vi "Get Parameter.vi"(8 "error in (no error)":errorcluster, 11 "SolarSystems M266 in":refnum<class "SolarSystems M266.lvclass">) -> (0 "error out":errorcluster, 2 "Parameter":refnum<class "AbstractData.lvclass">, 3 "SolarSystems M266 out":refnum<class "SolarSystems M266.lvclass">)   [LabVIEW 2014, in "SolarSystems M266.lvclass"]
uses:
  SolarSystems M266.lvclass
  Framework/Model/Data/DataSingleElement/DataSingleElement.lvclass
  Framework/Model/Data/AbstractData/AbstractData.lvclass
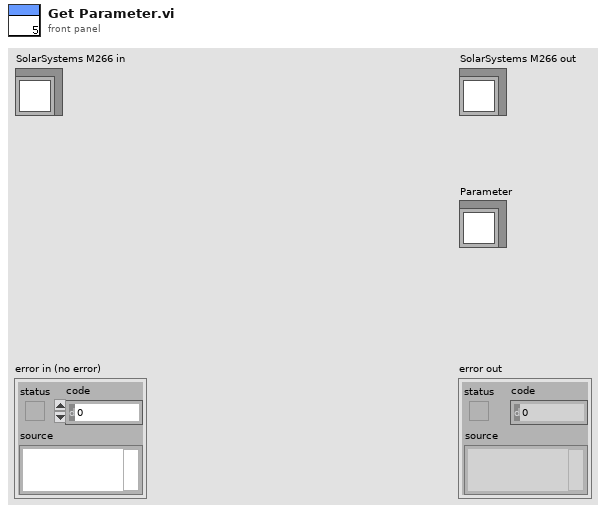
[diagram p1: front panel]
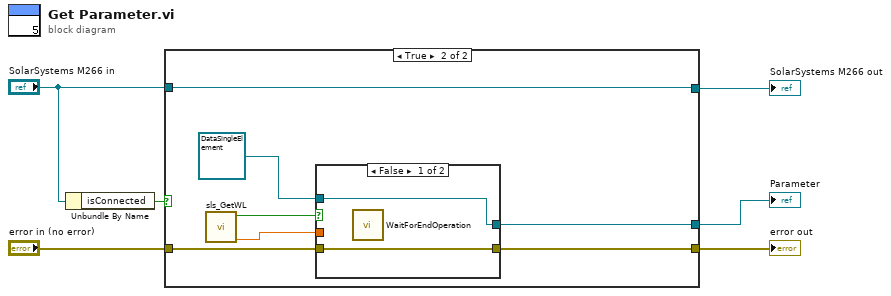
[diagram p0: block diagram]
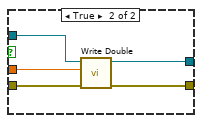
[diagram p3: hidden frame]
diagram:
  n1 = Unbundle By Name("SolarSystems M266 in") -> ("isConnected"=w4:bool)
  n2 = case shown="True" w4 {
    tunnel: [w7 w12] -> w6
    tunnel: "error in (no error)" -> [w7 w13]
    tunnel: [w8 w15] -> w2
    tunnel: "SolarSystems M266 in" -> [w8 w15]
    tunnel: [_ w14] -> w1
    frame False {
    }
    frame True {
      n3 = call "sls_GetWL.vi"() -> ("Current WL"=w10:dbl, "Result"=w11:bool)  [unwired: 10 in]
      n4 = case shown="False" w11 {
        tunnel: [w16 w22] -> w14
        tunnel: w13 -> [w17 w21]
        tunnel: [w17 w20] -> w12
        tunnel: w10 -> [_ w19]
        tunnel: refnum<class "DataSingleElement.lvclass"> refnum ("DataSingleElement.lvclass") -> [w16 w18]
        frame False {
          n5 = call "WaitForEndOperation.vi"() -> ()  [unwired: 1 out]
        }
        frame True {
          n6 = call "Write Double.vi"("error in (no error)"=w21, "value"=w19, "DataSingleElement in"=w18) -> ("error out"=w20:errorcluster, "DataSingleElement out"=w22:refnum<class "DataSingleElement.lvclass">)  [unwired: 7 in]
        }
      }
    }
  }
  "error out" <- w6
  "SolarSystems M266 out" <- w2
  "Parameter" <- w1
